vi "Read-frameQ.vi"(8 "error in (no error)":errorcluster, 11 "dbc in":refnum<class "bFrameIO.lvclass">) -> (0 "error out":errorcluster, 2 "frameQ":refnum<queue>, 3 "dbc out":refnum<class "bFrameIO.lvclass">)   [LabVIEW 2015, in "bFrameIO.lvclass"]
uses:
  bFrameIO.lvclass
  <vilib>/xnet/xnet.llb/XNET Frame CAN.ctl
  <vilib>/xnet/xnet.llb/XNET Frame Type CAN.ctl
  bFrameIO.lvclass/bFrameIO.ctl
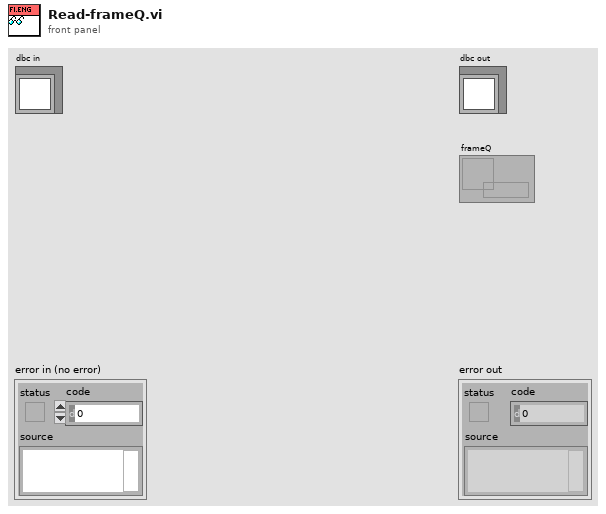
[diagram p1: front panel]
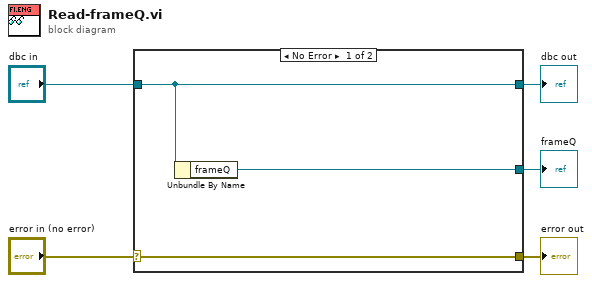
[diagram p0: block diagram]
diagram:
  n1 = case shown="No Error" "error in (no error)" {
    selector: "error in (no error)" -> [w8 w9]
    tunnel: [w8 w9] -> w4
    tunnel: [w7 w10] -> w2
    tunnel: "dbc in" -> [w7 w10]
    tunnel: [w6 _] -> w1
    frame No Error {
      n2 = Unbundle By Name(w7) -> ("frameQ"=w6:refnum<queue>)
    }
    frame Error {
    }
  }
  "error out" <- w4
  "dbc out" <- w2
  "frameQ" <- w1
